vi "Read Waveform Osciloscope.vi"(8 "error in (no error)":errorcluster, 10 "ReadWaveform":T1={"TEKTRONIX READ-WAVEFORM 2"={"Source (0: Channel 1)"=0, "Timeout (10000 ms) 2"=10000}, "EDU-X-1200A- READ-WAVEFORM"={"Bind Source Channel (2: None)"=2, "Timeout (10000 ms)"=10000, "Source Channel (0: Channel 1)"=0}} {"EDU-X-1200A- READ-WAVEFORM"."Source Channel (0: Channel 1)" items=["Channel 1"=0, "Channel 2"=1, "Channel 3"=2, "Channel 4"=3, "Waveform Memory 1"=5, "Waveform Memory 2"=6, "Serial Bus 1"=7, "Serial Bus 2"=8, "Digital Bus Low"=9, "Digital Bus High "=10, "Digital Bus 1"=11, "Digital Bus 2"=12, "External"=29, "Function 1"=32, "Function 2"=33, "Function 3"=34, "Function 4"=35, "Math 1"=36, "Math 2"=37, "Math 3"=38, "Math 4"=39, "FFT"=40, "Analog Bus"=41]; "EDU-X-1200A- READ-WAVEFORM"."Bind Source Channel (2: None)" items=["Sub Source 0", "Sub Source 1", "None"]; "TEKTRONIX READ-WAVEFORM 2"."Source (0: Channel 1)" items=["Channel 1", "Channel 2", "Channel 3", "Channel 4", "Math", "Reference A", "Reference B", "Reference C", "Reference D", "FFT"]}, 11 "Tektronicks in":refnum<class "Tektronicks.lvclass">) -> (0 "error out":errorcluster, 2 "Waveform Data":waveform(dbl)(graph), 3 "Tektronicks out":refnum<class "Tektronicks.lvclass">)   [LabVIEW 2020, in "Tektronicks.lvclass"]
uses:
  Tektronicks.lvclass
  TypeDefs/ReadWaveform--cluster.ctl
  Tektronicks.lvclass/Tektronicks.ctl
  <instrlib>/Tektronix TDS 200 1000 2000 Series/Tektronix TDS 200 1000 2000 Series.lvlib
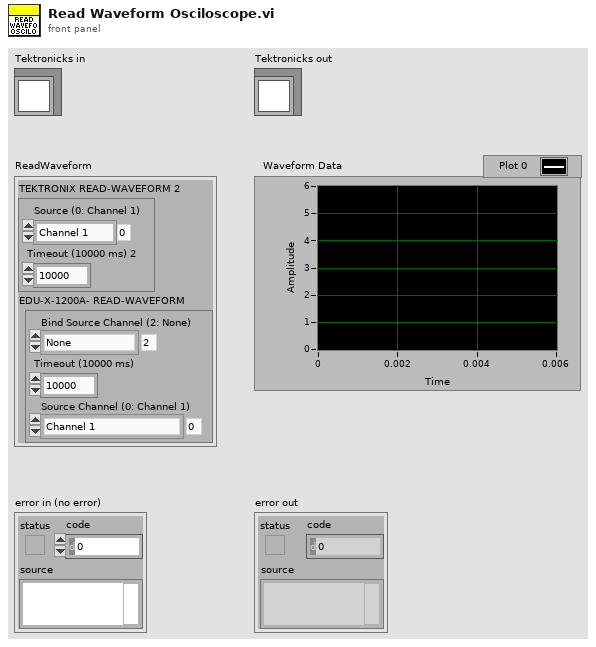
[diagram p1: front panel]
types:
  T1 = typedef "ReadWaveform--cluster.ctl" = cluster{"TEKTRONIX READ-WAVEFORM 2":cluster{"Source (0: Channel 1)":u16, "Timeout (10000 ms) 2":u32}, "EDU-X-1200A- READ-WAVEFORM":cluster{"Bind Source Channel (2: None)":i32, "Timeout (10000 ms)":u32, "Source Channel (0: Channel 1)":i32}}
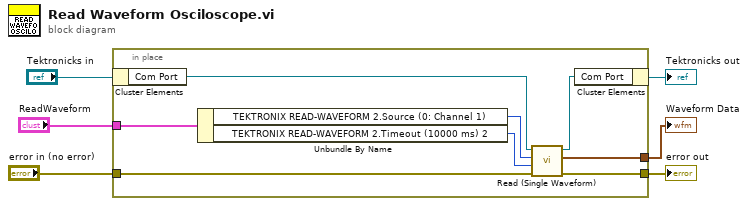
[diagram p0: block diagram]
diagram:
  n1 = in-place {
    in-place-border: "error in (no error)" -> [w12]
    in-place-border: [w11] -> w3
    in-place-border: [w10] -> w2
    in-place-border: "ReadWaveform" -> [w9]
    n2 = in-place-cluster #1("Tektronicks in") -> ("Com Port"=w14:refnum<visa-resource-name>)
    n3 = Unbundle By Name(w9) -> ("TEKTRONIX READ-WAVEFORM 2.Source (0: Channel 1)"=w8:u16, "TEKTRONIX READ-WAVEFORM 2.Timeout (10000 ms) 2"=w7:u32)
    n4 = call <instrlib>:"Read (Single Waveform).vi"("error in (no error)"=w12, "Timeout (10000 ms)"=w7, "Source (0: Channel 1)"=w8, "VISA resource name"=w14) -> ("error out"=w11:errorcluster, "Waveform Data"=w10:waveform(dbl), "VISA resource name out"=w13:refnum<visa-resource-name>)  [unwired: 5 in]
    n5 = in-place-cluster #1("Com Port"=w13) -> (→"Tektronicks out":refnum<class "Tektronicks.lvclass">)
  }
  "error out" <- w3
  "Waveform Data" <- w2
